vi "Create Events Table_Beltwatch.vi"() -> ()   [LabVIEW 2017, in "Beltwatch SQLite.lvlib"]
uses:
  Database/Beltwatch SQLite.lvlib
  Common64/Database/SQ Lite/SQ Lite Cluster Action.ctl
panel:
  out "source":string
  in  "Pre String":string="DROP TABLE IF EXISTS events;\n\n\nCREATE TABLE events (\n  db_id INTEGER PRIMARY KEY AUTOINCREMENT"
  in  "Readingse":T1[](array[typedef])=[{"Include"=TRUE, "Name"="Reading #", "SQLite3 type"=enum."SQLITE_INTEGER"}, {"Include"=TRUE, "Name"="Readings", "SQLite3 type"=enum."SQLITE3_TEXT"}, {"Include"=TRUE, "Name"="Reading Name", "SQLite3 type"=enum."SQLITE3_TEXT"}, {"Include"=TRUE, "Name"="TypeVal", "SQLite3 type"=enum."SQLITE_INTEGER"}, {"Include"=TRUE, "Name"="Alarm priority", "SQLite3 type"=enum."SQLITE_INTEGER"}, {"Include"=FALSE, "Name"="Display precision", "SQLite3 type"=enum."undefined type (0)"}, {"Include"=TRUE, "Name"="TypeStr", "SQLite3 type"=enum."SQLITE3_TEXT"}, {"Include"=TRUE, "Name"="AlarmPriorityStr", "SQLite3 type"=enum."SQLITE3_TEXT"}]
  out "?":errorcluster
  out "String":string
  out "SQLite3 type":T2(ring)
  in  "Events":T1[](array[typedef])=[{"Include"=TRUE, "Name"="Position", "SQLite3 type"=enum."SQLITE_INTEGER"}, {"Include"=TRUE, "Name"="Event Type", "SQLite3 type"=enum."SQLITE_INTEGER"}, {"Include"=TRUE, "Name"="Area", "SQLite3 type"=enum."SQLITE_INTEGER"}, {"Include"=TRUE, "Name"="Channels", "SQLite3 type"=enum."SQLITE_INTEGER"}, {"Include"=TRUE, "Name"="Start position", "SQLite3 type"=enum."SQLITE_INTEGER"}, {"Include"=TRUE, "Name"="End  position", "SQLite3 type"=enum."SQLITE_INTEGER"}, {"Include"=TRUE, "Name"="Name", "SQLite3 type"=enum."SQLITE3_TEXT"}, {"Include"=TRUE, "Name"="Offset", "SQLite3 type"=enum."SQLITE_INTEGER"}, {"Include"=TRUE, "Name"="Length", "SQLite3 type"=enum."SQLITE_INTEGER"}, {"Include"=TRUE, "Name"="Action marker", "SQLite3 type"=enum."SQLITE3_TEXT"}, {"Include"=TRUE, "Name"="Event", "SQLite3 type"=enum."SQLITE_INTEGER"}, {"Include"=TRUE, "Name"="# Defects", "SQLite3 type"=enum."SQLITE_INTEGER"}, {"Include"=TRUE, "Name"="jpg Image", "SQLite3 type"=enum."SQLITE_BLOB"}, {"Include"=TRUE, "Name"="chan maxs", "SQLite3 type"=enum."SQLITE_INTEGER"}, {"Include"=TRUE, "Name"="chan mins", "SQLite3 type"=enum."SQLITE_INTEGER"}, {"Include"=TRUE, "Name"="TimeStamp", "SQLite3 type"=enum."SQLITE_INTEGER"}, {"Include"=TRUE, "Name"="Readings", "SQLite3 type"=enum."SQLITE_INTEGER"}, {"Include"=TRUE, "Name"="ID", "SQLite3 type"=enum."SQLITE_INTEGER"}, {"Include"=TRUE, "Name"="New", "SQLite3 type"=enum."SQLITE_INTEGER"}, {"Include"=TRUE, "Name"="Hires Track", "SQLite3 type"=enum."SQLITE_INTEGER"}, {"Include"=TRUE, "Name"="2D overlay", "SQLite3 type"=enum."SQLITE_INTEGER"}, {"Include"=TRUE, "Name"="update", "SQLite3 type"=enum."SQLITE_INTEGER"}, {"Include"=TRUE, "Name"="Field #", "SQLite3 type"=enum."SQLITE_INTEGER"}, {"Include"=TRUE, "Name"="Events Class", "SQLite3 type"=enum."SQLITE_INTEGER"}, {"Include"=TRUE, "Name"="Sync", "SQLite3 type"=enum."SQLITE_INTEGER"}, {"Include"=TRUE, "Name"="Insert Offset", "SQLite3 type"=enum."SQLITE_INTEGER"}, {"Include"=TRUE, "Name"="Next trend", "SQLite3 type"=enum."SQLITE_INTEGER"}, {"Include"=TRUE, "Name"="Speed", "SQLite3 type"=enum."SQLITE_INTEGER"}]
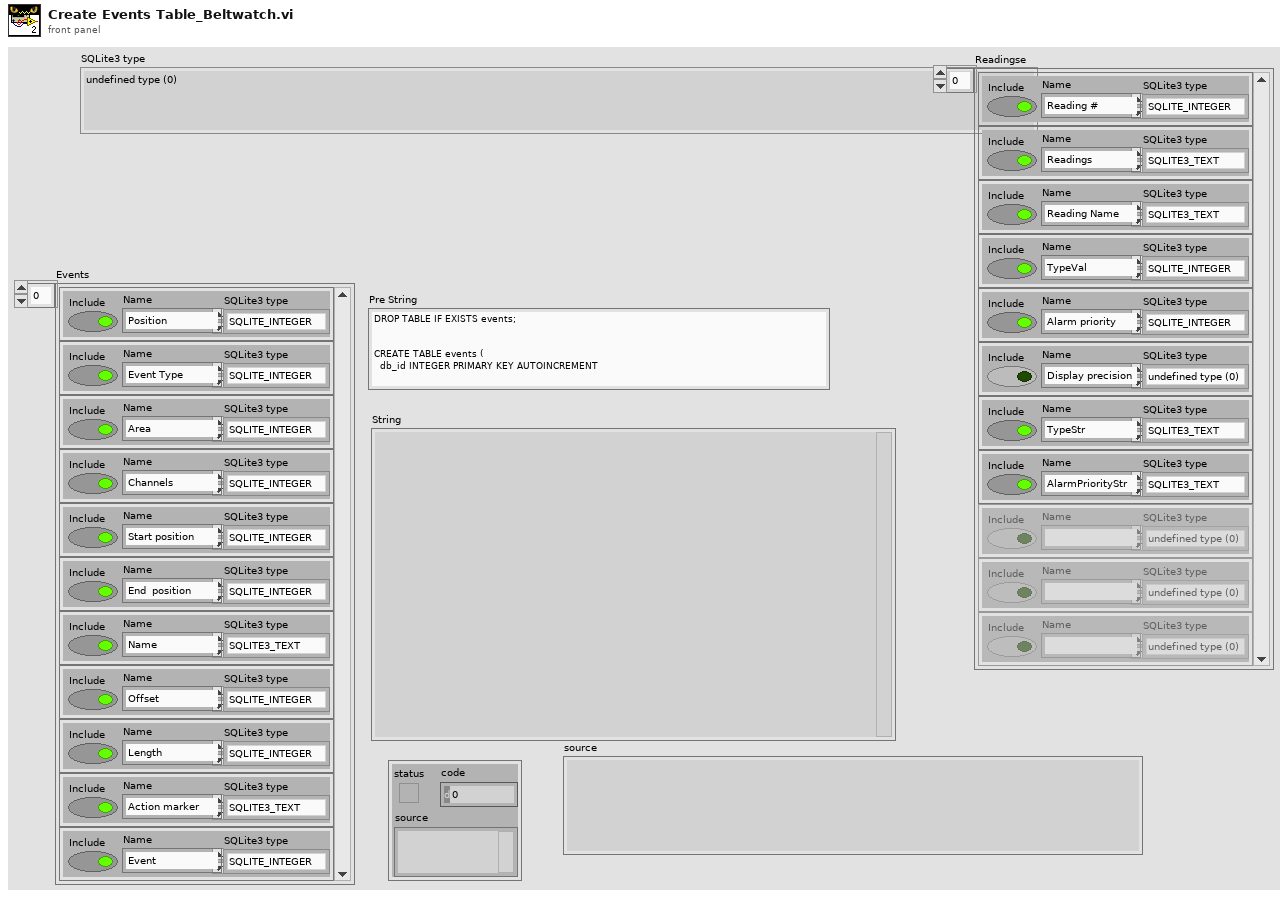
[diagram p1: front panel]
types:
  T1 = typedef "Beltwatch SQLite.lvlib/SQ Lite Cluster Action.ctl" = cluster{"Include":bool, "Name":string, "SQLite3 type":enum32{"undefined type (0)", "SQLITE_INTEGER", "SQLITE_FLOAT", "SQLITE3_TEXT", "SQLITE_BLOB", "SQLITE_NULL", "undefined type"}}
  T2 = enum32{"undefined type (0)", "SQLITE_INTEGER", "SQLITE_FLOAT", "SQLITE3_TEXT", "SQLITE_BLOB", "SQLITE_NULL", "undefined type"}
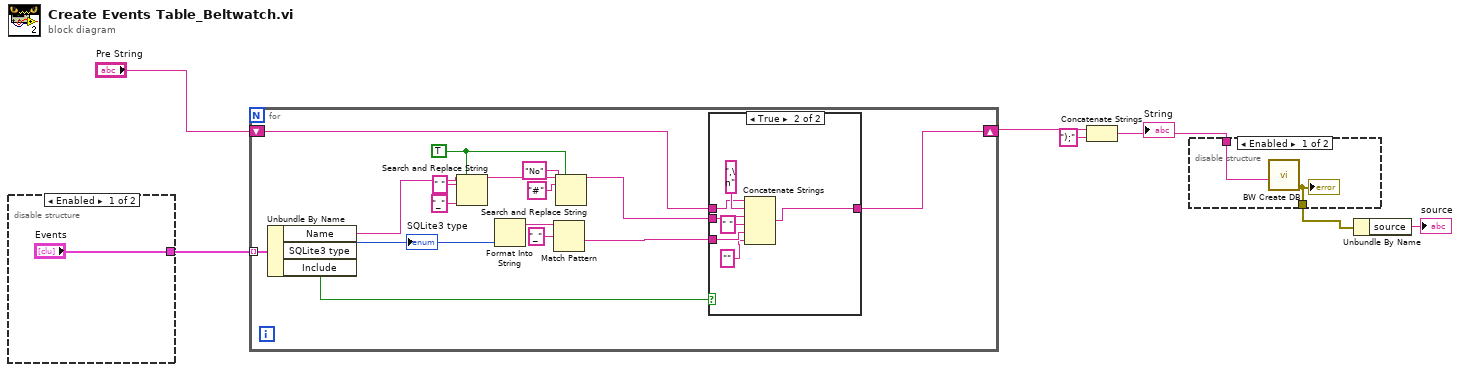
[diagram p0: block diagram]
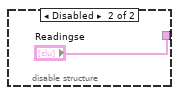
[diagram p2: hidden frame]
diagram:
  n1 = disable-structure shown="Enabled" {
    disable-tunnel: ["Events" "Readingse"] -> w6
    frame Enabled {
    }
    frame Disabled {
    }
  }
  n2 = for {
    shift-right: [w18] -> w5
    shift-left: "Pre String" -> [w25]
    tunnel: w6 -> [w24] mode=indexing
    w14 = TRUE ("replace all? (F)")
    n3 = Unbundle By Name(w24) -> ("Name"=w17:string, "SQLite3 type"=w22:T2, "Include"=w23:bool)
    "SQLite3 type" <- w22
    n4 = Search and Replace String(replace all?=w14, input string=w17, search string=" ", replace string="_" ("replace string (\"\")")) -> (result string=w13:string)  [unwired: 4 in, 3 out]
    n5 = Format Into String(w22) -> (resulting string=w21:string)  [unwired: 3 in, 1 out]
    n6 = Match Pattern(string=w21, regular expression="_") -> (after substring=w19:string)  [unwired: 1 in, 3 out]
    n7 = Search and Replace String(replace all?=w14, input string=w13, search string="#" ("replace string (\"\")"), replace string="No" ("replace string (\"\")")) -> (result string=w10:string)  [unwired: 4 in, 3 out]
    n8 = case shown="True" w23 {
      tunnel: w25 -> [w26 w28]
      tunnel: w10 -> [_ w33]
      tunnel: w19 -> [_ w31]
      tunnel: [w26 w30] -> w18
      frame False {
      }
      frame True {
        n9 = Concatenate Strings(w28, ",\n" ("string"), w33, " " ("string"), w31, "" ("string")) -> (w30:string)
      }
    }
  }
  n10 = Concatenate Strings(w5, ");" ("string")) -> (w3:string)
  "String" <- w3
  n11 = disable-structure shown="Enabled" {
    disable-tunnel: w3 -> [w35 _]
    disable-tunnel: [w34 _] -> w2
    frame Enabled {
      n12 = call "BW Create DB.vi"("String"=w35) -> ("error out"=w34:errorcluster)  [unwired: 10 in]
      "?" <- w34
    }
    frame Disabled {
    }
  }
  n13 = Unbundle By Name(w2) -> ("source"=→"source":string)
